vi "ClusterOperations.vi"() -> ()   [LabVIEW 2015]
panel:
  in  "Cluster Control":T1
  out "Cluster Indicadores":T2 {"Gauge" scale=0.0..50.0; "Tanque" scale=0.0..30.0; "Termometro" scale=0.0..50.0}
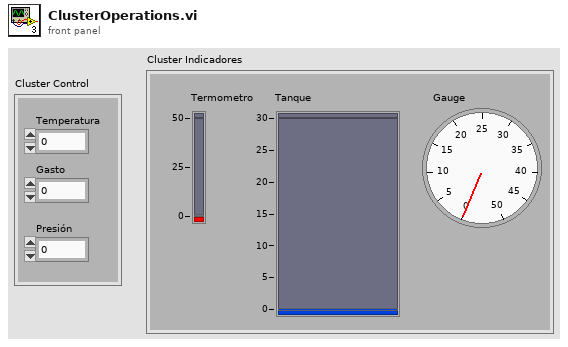
[diagram p1: front panel]
types:
  T1 = cluster{"Temperatura":dbl, "Gasto":dbl, "Presión":dbl}
  T2 = cluster{"Termometro":dbl, "Tanque":dbl, "Gauge":dbl}
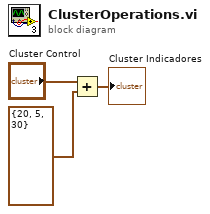
[diagram p0: block diagram]
diagram:
  n1 = Add(x="Cluster Control", y=cluster{i32, i32, i32} {20, 5, 30}) -> (x+y=→"Cluster Indicadores":cluster{dbl, dbl, dbl})
